vi "逆解算法.vi"() -> ()   [LabVIEW 2023]
panel:
  in  "y":dbl
  out "theta2":dbl
  out "theta1":dbl
  in  "簇":cluster{"数值":dbl, "数值 2":dbl}
  in  "x":dbl
  in  "函数名称":string="inverse_kinematics"
  in  "模块路径":path
  in  "错误输入（无错误）":errorcluster
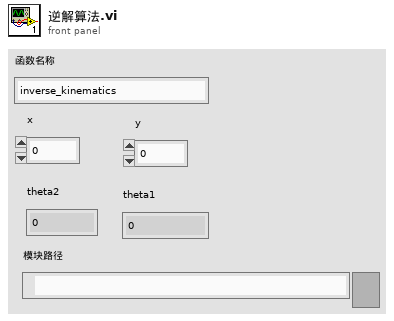
[diagram p1: front panel]
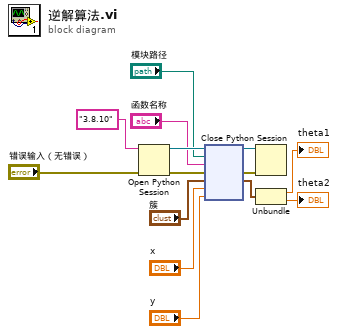
[diagram p0: block diagram]
diagram:
  n1 = Open Python Session(python version="3.8.10" ("Python版本"), 3:"错误输入（无错误）") -> (session out=w14:refnum<k35>, error out=w13:errorcluster)  [unwired: 1 in]
  n2 = node(w14, "模块路径", "函数名称", w13, "簇", "x", "y") -> (w11:refnum<k35>, w12:errorcluster, w5:cluster{"数值":dbl, "数值 2":dbl})  [unwired: 2 in, 2 out]
  n3 = Close Python Session(session in=w11, error in=w12) -> ()  [unwired: 1 out]
  n4 = Unbundle(w5) -> ("数值"=→"theta1":dbl, "数值 2"=→"theta2":dbl)
